vi "M09 Hydro pool.vi"(11 "EV3 in":T1) -> (3 "NXT/EV3":T1)   [LabVIEW 2016]
uses:
  <vilib>/NXT/Subs/LVHSConnector.ctl
  <vilib>/NXT/LegoClasses/BrickReference/BrickReference.lvclass
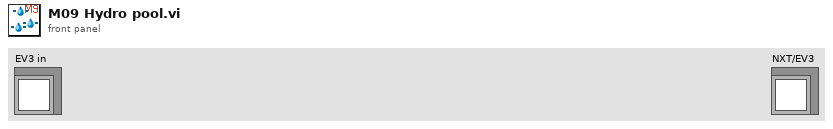
[diagram p1: front panel]
types:
  T1 = typedef "LVHSConnector.ctl" = refnum<class "BrickReference.lvclass">
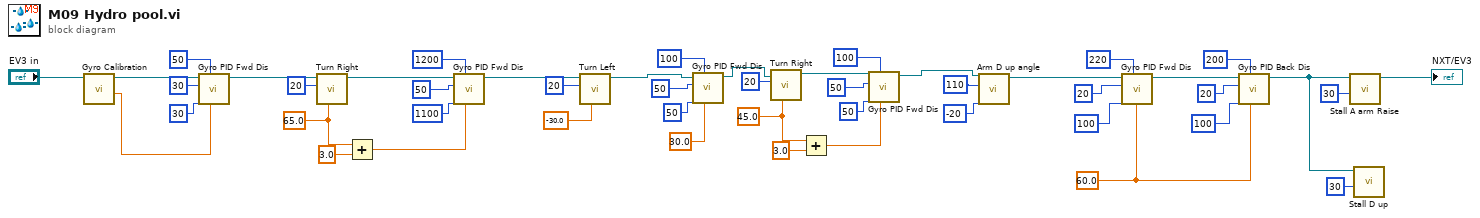
[diagram p0: block diagram]
diagram:
  w9 = sgl 45.0 ("Turning angle")
  w30 = sgl 60.0 ("Target angle")
  w22 = sgl 65.0 ("Turning angle")
  n1 = call "Gyro Calibration.vi"("NXT/EV3"="EV3 in") -> ("Degrees"=w23:sgl, "NXT/EV3"=w24:T1)  [unwired: 6 in, 1 out]
  n2 = call "Gyro PID Fwd Dis.vi"("Target angle"=w23, "Threshold to stop"=50, "Threshold to slow"=30, "Max. speed"=30, "EV3 in"=w24) -> ("EV3 out"=w44:T1)  [unwired: 6 in]
  n3 = call "Turn Right.vi"("Turning angle"=w22, "Motor B (right)"=i8 20, "EV3 in"=w44) -> ("EV3 out"=w39:T1)  [unwired: 8 in]
  n4 = Add(x=w22, y=sgl 3.0) -> (x+y=w20:sgl)
  n5 = call "Gyro PID Fwd Dis.vi"("Target angle"=w20, "Threshold to stop"=1200, "Threshold to slow"=1100, "Max. speed"=50, "EV3 in"=w39) -> ("EV3 out"=w26:T1)  [unwired: 6 in]
  n6 = call "Turn Left.vi"("Turning angle"=sgl -30.0, "Motor B (right)"=i8 20, "EV3 in"=w26) -> ("EV3 out"=w13:T1)  [unwired: 8 in]
  n7 = call "Gyro PID Fwd Dis.vi"("Target angle"=sgl 30.0, "Threshold to stop"=100, "Threshold to slow"=50, "Max. speed"=50, "EV3 in"=w13) -> ("EV3 out"=w7:T1)  [unwired: 6 in]
  n8 = call "Turn Right.vi"("Turning angle"=w9, "Motor B (right)"=i8 20, "EV3 in"=w7) -> ("EV3 out"=w3:T1)  [unwired: 8 in]
  n9 = Add(x=w9, y=sgl 3.0) -> (x+y=w1:sgl)
  n10 = call "Gyro PID Fwd Dis.vi"("Target angle"=w1, "Threshold to stop"=100, "Threshold to slow"=50, "Max. speed"=50, "EV3 in"=w3) -> ("EV3 out"=w2:T1)  [unwired: 6 in]
  n11 = call "Arm D up angle.vi"("Power"=i8 -20, "Rotation"=110, "EV3 in"=w2) -> ("EV3 out"=w33:T1)  [unwired: 8 in]
  n12 = call "Gyro PID Fwd Dis.vi"("Target angle"=w30, "Threshold to stop"=220, "Threshold to slow"=100, "Max. speed"=20, "EV3 in"=w33) -> ("EV3 out"=w32:T1)  [unwired: 6 in]
  n13 = call "Gyro PID Back Dis.vi"("Target angle"=w30, "Threshold to stop"=200, "Threshold to slow"=100, "Max. speed"=20, "EV3 in"=w32) -> ("EV3 out"=w19:T1)  [unwired: 6 in]
  n14 = call "Stall A arm Raise.vi"("Power"=i8 30, "NXT/EV3"=w19) -> ("NXT/EV3"=→"NXT/EV3":T1)  [unwired: 9 in]
  n15 = call "Stall D up.vi"("Power"=i8 30, "NXT/EV3"=w19) -> ()  [unwired: 9 in, 1 out]
